vi "R1pHControl_SetParams.vi"(7 "LabVIEW Web Service Request":refnum<class "Web Request.lvclass">) -> (2 "ControlStatus":string, 3 "pH_SetParams_Out":T1)   [LabVIEW 2016]
uses:
  <vilib>/wsapi/Web Request.lvclass
  Controls/pH_SetParams Standard.ctl
panel:
  in  "Pump Time On, secs":dbl
  in  "Tolerance":dbl
  in  "Set Point":dbl
  # "Use the Web Service Request input terminal to call the VIs on the Web Services palette. Do not remove it from the connector pane unless you don't need access to the palette."
  # "Each additional control wired to the connector pane will be available as an input in the URL. To include an indicator in terminal-mode output (the default setting), it must also be wired to the connector pane."
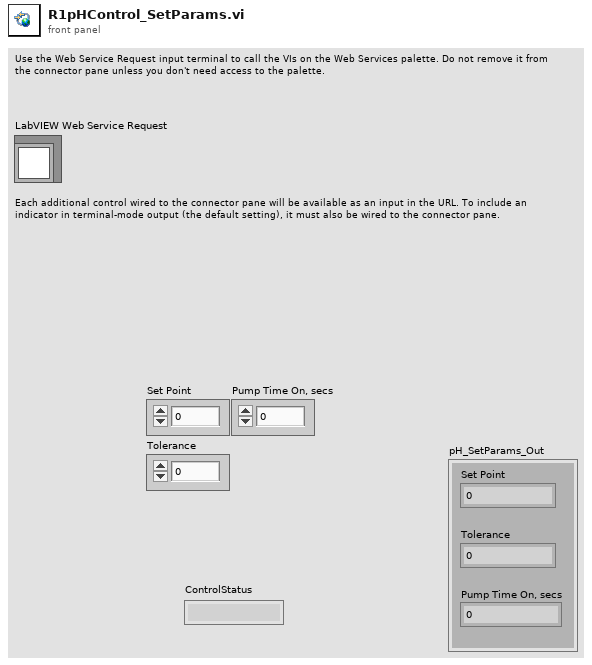
[diagram p1: front panel]
types:
  T1 = typedef "pH_SetParams Standard.ctl" = cluster{"Set Point":dbl, "Tolerance":dbl, "Pump Time On, secs":dbl}
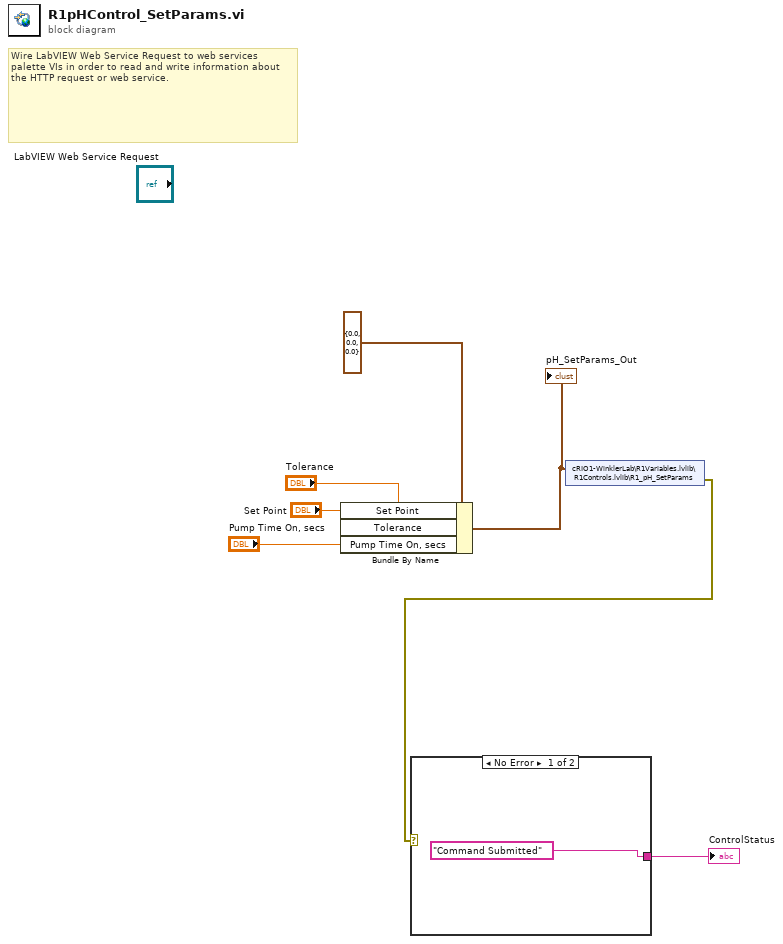
[diagram p0: block diagram]
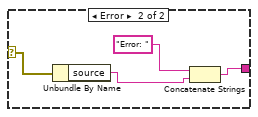
[diagram p2: hidden frame]
diagram:
  # "Wire LabVIEW Web Service Request to web services palette VIs in order to read and write information about the HTTP request or web service."
  n1 = Bundle By Name(cluster=T1 {"Set Point"=0.0, "Tolerance"=0.0, "Pump Time On, secs"=0.0} ("R1_pH_SetParams"), "Set Point"="Set Point", "Tolerance"="Tolerance", "Pump Time On, secs"="Pump Time On, secs") -> (w1:T1)
  "pH_SetParams_Out" <- w1
  n2 = shared-variable "cRIO1-WinklerLab\\R1Variables.lvlib\\R1Controls.lvlib\\R1_pH_SetParams"(w1) -> (error out=w5:errorcluster)  [unwired: 1 in]
  n3 = case shown="No Error" w5 {
    selector: w5 -> [_ w10]
    tunnel: ["Command Submitted" ("ControlStatus") w9] -> w7
    frame No Error {
    }
    frame Error {
      n4 = Unbundle By Name(w10) -> ("source"=w11:string)
      n5 = Concatenate Strings("Error: ", w11) -> (w9:string)
    }
  }
  "ControlStatus" <- w7
